vi "Merge Waveform.vi"(6 "Digital":bool, 8 "Error":errorcluster, 9 "Waveform To Append":T1, 11 "WavBuf":refnum<class "WavBuf.lvclass">) -> (0 "Error Out":errorcluster, 3 "WavBuf Out":refnum<class "WavBuf.lvclass">)   [LabVIEW 2020, in "WavBuf.lvclass"]
uses:
  WavBuf.lvclass
  Universal Controls/Waveform_Data.ctl
  WavBuf.lvclass/WavBuf.ctl
  Support/Waveform_Resample with new dt.vi
  Support/Wavform_Select dt and check valid time.vi
  Support/t0_Valid.vi
  Support/tf_from t0.vi
  Support/t0_from tf.vi
  Support/Waveform_Read Write End Point Index.vi
  Support/Dbl Array_Linearize NAN values.vi
  Support/Timestamp_Convert Difference to dt Increments.vi
  <vilib>/Waveform/WDTOps.llb/Check for Equality.vi
  <vilib>/Waveform/WDTOps.llb/Waveform Duration.vi
  <vilib>/Waveform/WDTOps.llb/WDT Waveform Duration DBL.vi
  Support/Dbl Array_Place Line between points.vi
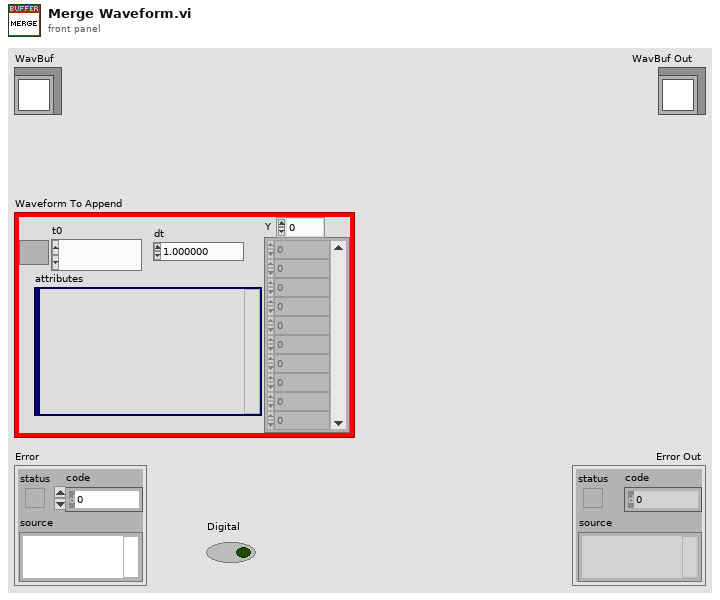
[diagram p1: front panel]
types:
  T1 = typedef "Waveform_Data.ctl" = waveform(dbl)
  T2 = enum16{"Combine Times", "Keep Waveform Size", "Set to Size Value", "Set to Time(S) Value"}
  T3 = typedef "Ref_DVR_Buffer.ctl" = refnum<data-value>
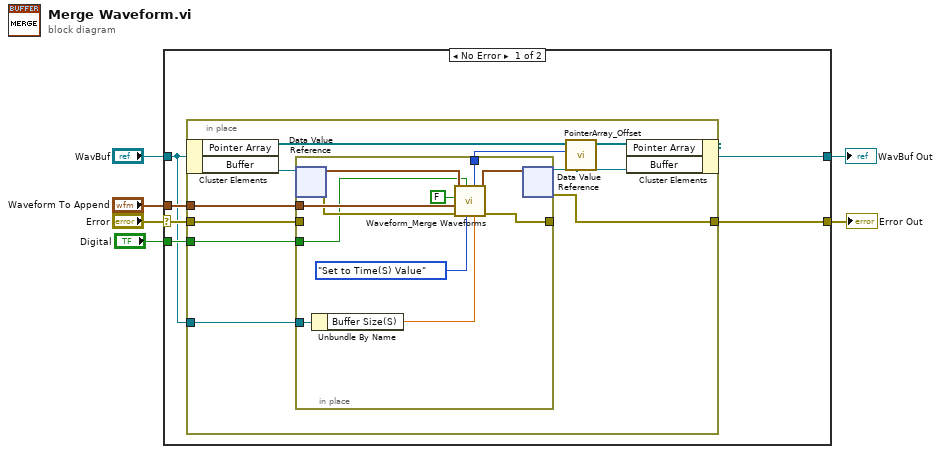
[diagram p0: block diagram]
diagram:
  n1 = case shown="No Error" "Error" {
    selector: "Error" -> [w11 w35]
    tunnel: [w9 w35] -> w5
    tunnel: [w12 w34] -> w3
    tunnel: "WavBuf" -> [w7 w34]
    tunnel: "Waveform To Append" -> [w10 _]
    tunnel: "Digital" -> [w8 _]
    frame No Error {
      n2 = in-place {
        in-place-border: w11 -> [w22]
        in-place-border: [w15] -> w9
        in-place-border: w10 -> [w21]
        in-place-border: w8 -> [w14]
        in-place-border: w7 -> [w13]
        n3 = in-place-cluster #1(w7) -> ("Pointer Array"=w17:refnum<class "_Pointer.lvclass">[], "Buffer"=w20:T3)
        n4 = in-place {
          in-place-border: w22 -> [_]
          in-place-border: [w28] -> _
          in-place-border: [w33] -> w18
          in-place-border: w21 -> [w31]
          in-place-border: w14 -> [w27]
          in-place-border: w13 -> [w24]
          n5 = in-place-dvr #2(w20) -> (w32:T1, w30:errorcluster)
          n6 = Unbundle By Name(w24) -> ("Buffer Size(S)"=w23:dbl)
          n7 = call "Waveform_Merge Waveforms.vi"("Size or Time(S)"=w23, "Size Select"=T2."Set to Time(S) Value", "Digital"=w27, "Error"=w30, "Waveform To Merge"=w31, "Use Merge Dt"=FALSE, "Waveform"=w32) -> ("Error Out"=w28:errorcluster, "Waveform Out"=w29:T1, "Offset Out"=w33:i32)  [unwired: 1 in, 1 out]
          n8 = in-place-dvr #2(w29) -> (w19:T3, w15:errorcluster)
        }
        n9 = call "PointerArray_Offset.vi"("Buffer"=w19, "Total Starting Offset"=w18, "Pointer Array"=w17) -> ("Pointer Array Out"=w16:refnum<class "_Pointer.lvclass">[])  [unwired: 8 in]
        n10 = in-place-cluster #1("Pointer Array"=w16, "Buffer"=w19) -> (w12:refnum<class "WavBuf.lvclass">)
      }
    }
    frame Error {
    }
  }
  "Error Out" <- w5
  "WavBuf Out" <- w3
